vi "Get_Rotation_Centre.vi"() -> ()   [LabVIEW 2011]
uses:
  <vilib>/Math Plots/3D Math Plots/3D Scatter/3D Scatter XCtrl/3D Scatter.xctl
  <vilib>/Math Plots/3D Math Plots/3D Scatter/3D Scatter Datatype/Public/Plot Helper (Vector).vi
  <vilib>/Math Plots/3D Math Plots/3D Scatter/3D Scatter Datatype/3D Scatter Datatype.lvclass
  <vilib>/gmath/NI_Gmath.lvlib
panel:
  in  "Pivot Axis":u16(ring) items=["Z axis (Yaw)", "Y axis (Pitch)", "X axis (Roll)"]
  out "r":dbl format="%.2f"
  out "x0, y0, z0":dbl[](array[numeric]) format="%.2f"
  in  "Point Cloud":cluster{"X":dbl, "Y":dbl, "Z":dbl}[](array[cluster])
  out "3D Scatter":refnum<class "3D Plot Datatype.lvclass">[](xcontrol)
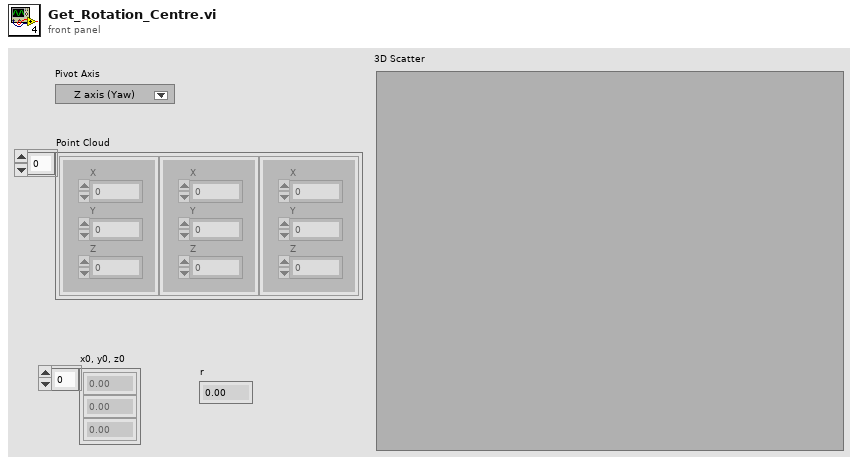
[diagram p1: front panel]
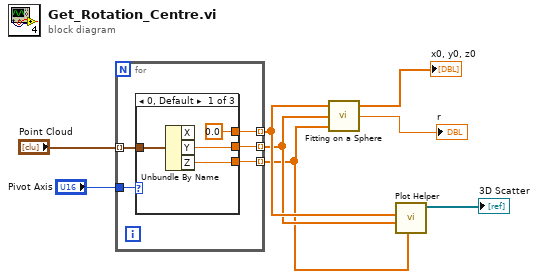
[diagram p0: block diagram]
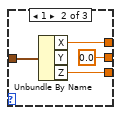
[diagram p2: hidden frame]
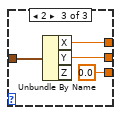
[diagram p3: hidden frame]
diagram:
  n1 = for {
    tunnel: "Point Cloud" -> [w13] mode=indexing
    tunnel: [w12] -> w6 mode=indexing
    tunnel: [w11] -> w5 mode=indexing
    tunnel: [w10] -> w4 mode=indexing
    tunnel: "Pivot Axis" -> [w9]
    n2 = case shown="0, Default" w9 {
      tunnel: w13 -> [w17 w21 w25]
      tunnel: [0.0 ("X") w20 w24] -> w12
      tunnel: [w16 0.0 ("Y") w23] -> w11
      tunnel: [w15 w19 0.0 ("Z")] -> w10
      frame 0, Default {
        n3 = Unbundle By Name(w17) -> ("Y"=w16:dbl, "Z"=w15:dbl)  [unwired: 1 out]
      }
      frame 1 {
        n4 = Unbundle By Name(w21) -> ("X"=w20:dbl, "Z"=w19:dbl)  [unwired: 1 out]
      }
      frame 2 {
        n5 = Unbundle By Name(w25) -> ("X"=w24:dbl, "Y"=w23:dbl)  [unwired: 1 out]
      }
    }
  }
  n6 = call <vilib>:"Fitting on a Sphere.vi"("Z"=w4, "Y"=w5, "X"=w6) -> ("r"=→"r":dbl, "x0, y0, z0"=→"x0, y0, z0":dbl[])  [unwired: 1 out]
  n7 = call-poly <vilib>:"Plot Helper.vi"("z vector"=w4, "y vector"=w5, "x vector"=w6) -> ("3D Plot lvclass Array out"=→"3D Scatter":refnum<class "3D Plot Datatype.lvclass">[])  [unwired: 3 in, 5 out]
